vi "Digital Write Multiple Channels.vi"(8 "error in (no error)":errorcluster, 9 "Values":bool[](array[boolean]), 10 "Indices":i32[](array[numeric]), 11 "NI-DAQ in":refnum<class "NI-DAQ.lvclass">) -> (0 "error out":errorcluster, 3 "NI-DAQ out":refnum<class "NI-DAQ.lvclass">)   [LabVIEW 2020, in "NI-DAQ.lvclass"]
uses:
  NI-DAQ.lvclass
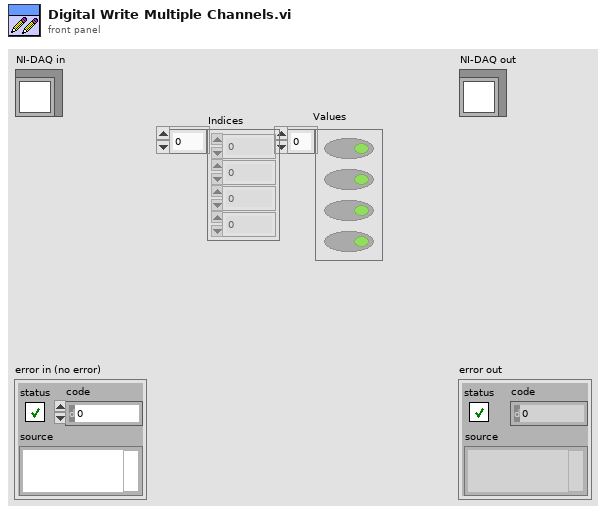
[diagram p1: front panel]
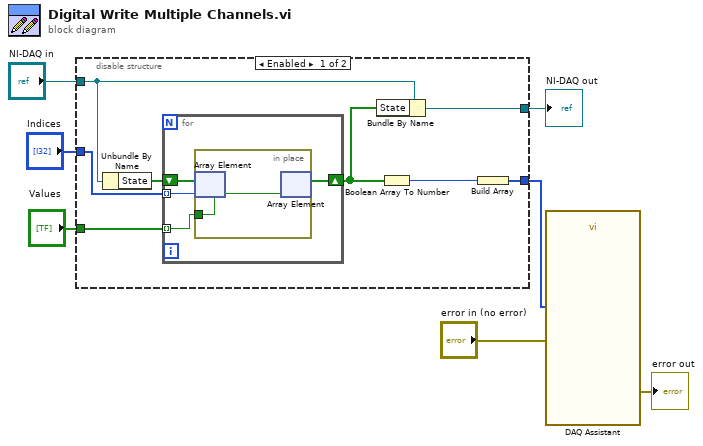
[diagram p0: block diagram]
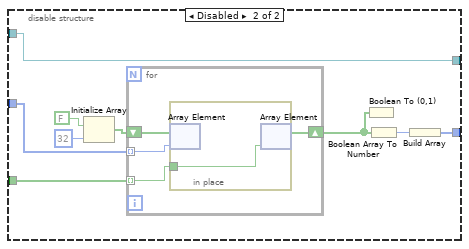
[diagram p2: hidden frame]
diagram:
  n1 = disable-structure shown="Enabled" {
    disable-tunnel: "NI-DAQ in" -> [w14 w29]
    disable-tunnel: [w13 w29] -> w6
    disable-tunnel: "Indices" -> [w10 w21]
    disable-tunnel: "Values" -> [w9 w22]
    disable-tunnel: [w8 w23] -> w2
    frame Enabled {
      n2 = Unbundle By Name(w14) -> ("State"=w12:bool[])
      n3 = for {
        tunnel: w9 -> [w19] mode=indexing
        tunnel: w10 -> [w18] mode=indexing
        shift-right: [w16] -> w11
        shift-left: w12 -> [w17]
        n4 = in-place {
          in-place-border: w19 -> [w20]
          n5 = in-place-array #1(w17, w18) -> ()  [unwired: 1 out]
          n6 = in-place-array #1(w20) -> (w16:bool[])  [unwired: 1 out]
        }
      }
      n7 = Bundle By Name(cluster=w14, "State"=w11) -> (w13:refnum<class "NI-DAQ.lvclass">)
      n8 = Boolean Array To Number(Boolean array=w11) -> (number=w15:u32)
      n9 = Build Array(w15) -> (w8:u32[])
    }
    frame Disabled {
      n10 = Initialize Array(FALSE, 32 ("dimension size")) -> (w28:bool[])
      n11 = for {
        tunnel: w21 -> [w33] mode=indexing
        tunnel: w22 -> [w32] mode=indexing
        shift-right: [w30] -> w25
        shift-left: w28 -> [w31]
        n12 = in-place {
          in-place-border: w32 -> [w34]
          n13 = in-place-array #2(w31, w33) -> ()  [unwired: 1 out]
          n14 = in-place-array #2(w34) -> (w30:bool[])  [unwired: 1 out]
        }
      }
      n15 = Boolean To (0,1)(Boolean=w25) -> ()  [unwired: 1 out]
      n16 = Boolean Array To Number(Boolean array=w25) -> (number=w24:u32)
      n17 = Build Array(w24) -> (w23:u32[])
    }
  }
  "NI-DAQ out" <- w6
  n18 = call "DAQ Assistant"("data"=w2, "error in"="error in (no error)") -> ("error out"=→"error out":errorcluster)  [unwired: 16 in, 1 out]
